vi "CFTS-Verify Acoustic Systems Dialog.vi"(0 "Expt State":T1, 2 "center on":refnum<vi>, 5 "Acoustic Systems":string[](array[string]), 7 "color":u32(colorbox)=16777216) -> (4 "Cluster out":T1, 8 "Canceled?":bool)   [LabVIEW 2020]
uses:
  CFTS-Experiment State.ctl
  epl-vi-lib/Utility VIs/Controls/KBackground Gradient/KBackground Gradient.xctl
panel:
  in  "background":dbl(xcontrol)
  in  "Left":u16(ring) items=[""=0, "ABI-L"=1, "ABI-R"=2, "Left"=3, "Right"=4, "SN24"=5, "SN31"=6, "SN32"=7, "SN36"=8, "SN40"=9, "SN41"=10, "SN42"=11, "Freefield"=12, "---"=65535]
  in  "Right":u16(ring) items=[""=0, "ABI-L"=1, "ABI-R"=2, "Left"=3, "Right"=4, "SN24"=5, "SN31"=6, "SN32"=7, "SN36"=8, "SN40"=9, "SN41"=10, "SN42"=11, "Freefield"=12, "---"=65535]
  in  "OK":bool
  # "Are these the acoustic systems you plan to use?\n\nIf not, select the correct ones before pressing OK."
  # "Acoustic Systems"
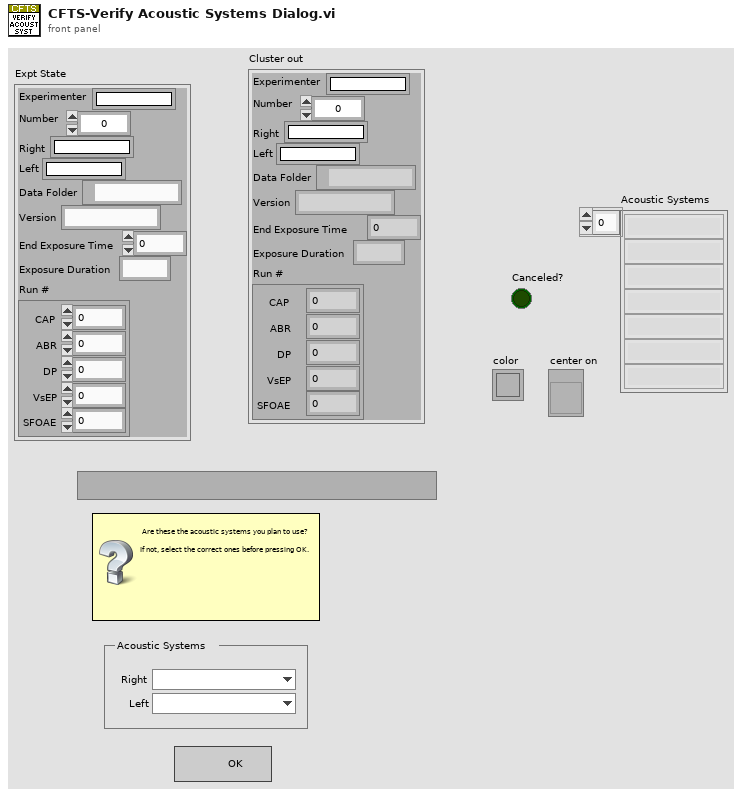
[diagram p1: front panel]
types:
  T1 = typedef "CFTS-Experiment State.ctl" = cluster{"Experimenter":string, "Number":u32, "Right":string, "Left":string, "Data Folder":path, "Version":string, "End Exposure Time":dbl, "Exposure Duration":string, "Run #":cluster{"CAP":i32, "ABR":i32, "DP":i32, "VsEP":i32, "SFOAE":i32}}
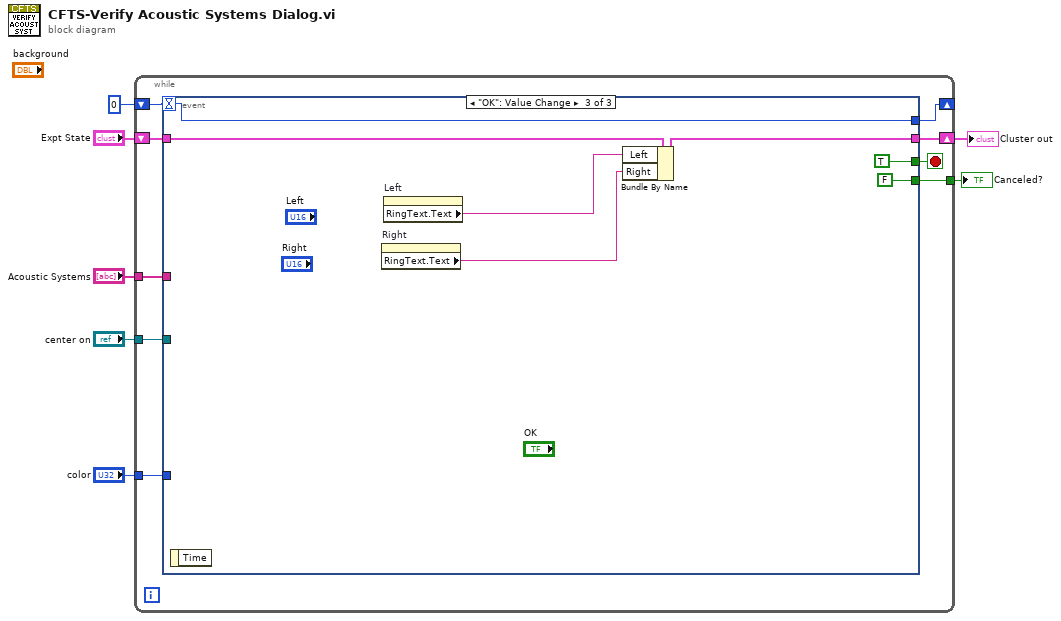
[diagram p0: block diagram]
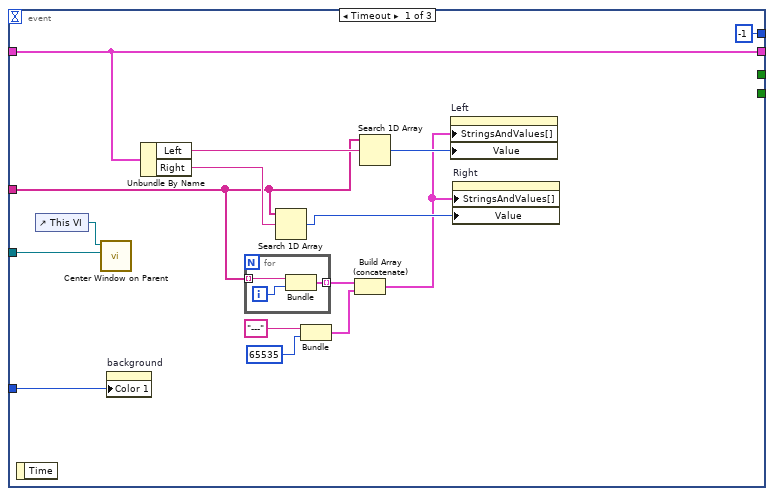
[diagram p2: hidden frame]
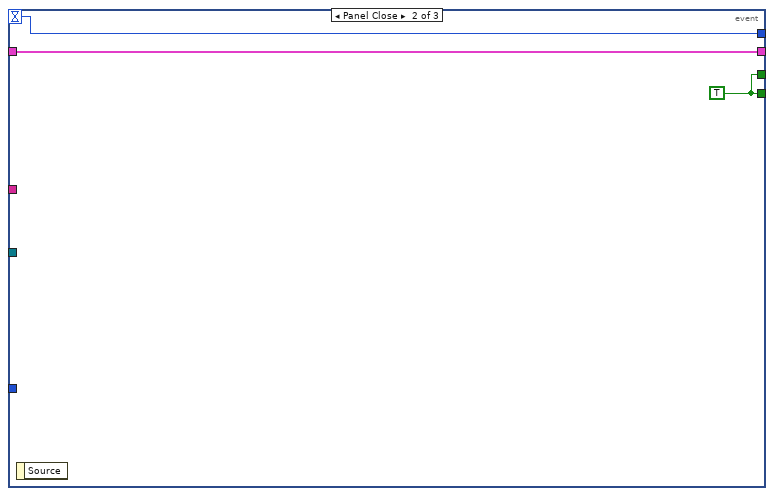
[diagram p3: hidden frame]
diagram:
  n1 = while {
    shift-right: [w15] -> _
    shift-left: 0 -> [w16]
    tunnel: [w12] -> w4
    shift-right: [w14] -> w5
    shift-left: "Expt State" -> [w11]
    tunnel: "center on" -> [w10]
    tunnel: "color" -> [w9]
    tunnel: "Acoustic Systems" -> [w8]
    stop <- w13 stop-if-true
    n2 = event shown="[2] \"OK\": Value Change" {
      selector: _ -> [_ _ _]
      dyn-events: _ -> [_ _ _]
      timeout: w16 -> [_ w37 w43]
      tunnel: [-1 w37 w43] -> w15
      tunnel: w11 -> [w21 w36 w44]
      tunnel: [w21 w36 w40] -> w14
      tunnel: [_ w35 TRUE] -> w13
      tunnel: [_ w35 FALSE] -> w12
      tunnel: w10 -> [w20 _ _]
      tunnel: w9 -> [w18 _ _]
      tunnel: w8 -> [w17 _ _]
      event Timeout {
        n3 = event-data() -> ()  [unwired: 1 in, 1 out]
        n4 = control-ref of="This VI"() -> (w19:refnum<vi>)
        n5 = call "Center Window on Parent.vi"("Parent VI"=w20, "VI in"=w19) -> ()  [unwired: 8 in, 2 out]
        n6 = property on="background" class="KBackground Gradient (strict)"("Color 1"=w18) -> ()  [unwired: 2 in, 2 out]
        n7 = Unbundle By Name(w21) -> ("Left"=w28:string, "Right"=w30:string)
        n8 = for {
          tunnel: w17 -> [w34] mode=indexing
          tunnel: [w32] -> w26 mode=indexing
          i -> [w33]
          n9 = Bundle("String"=w34, w33) -> (w32:cluster{"String":string, i32})  [unwired: 1 in]
        }
        n10 = Search 1D Array(1D array=w17, element=w30) -> (index of element=w29:i32)  [unwired: 1 in]
        n11 = Bundle("---", 65535) -> (w22:cluster{string, i32})  [unwired: 1 in]
        n12 = Build Array (concatenate)(w26, w22) -> (w23:cluster{"String":string, i32}[])
        n13 = Search 1D Array(1D array=w17, element=w28) -> (index of element=w27:i32)  [unwired: 1 in]
        n14 = property on="Left" class="Ring (strict)"("StringsAndValues[]"=w23, "Value"=w27) -> ()  [unwired: 2 in, 2 out]
        n15 = property on="Right" class="Ring (strict)"("StringsAndValues[]"=w23, "Value"=w29) -> ()  [unwired: 2 in, 2 out]
      }
      event Panel Close {
        w35 = TRUE
        n16 = event-data() -> ()  [unwired: 1 in, 1 out]
      }
      event "OK": Value Change {
        n17 = event-data() -> ()  [unwired: 1 in, 1 out]
        n18 = property on="Right" class="Ring (strict)"() -> ("RingText.Text"=w39:string)  [unwired: 2 in, 2 out]
        n19 = property on="Left" class="Ring (strict)"() -> ("RingText.Text"=w38:string)  [unwired: 2 in, 2 out]
        n20 = Bundle By Name(cluster=w44, "Left"=w38, "Right"=w39) -> (w40:T1)
      }
    }
  }
  "Cluster out" <- w5
  "Canceled?" <- w4
